vi "LC_Relay_main_WVM.vi"() -> ()   [LabVIEW 2016]
doc: "Reads relay data from FPGA layer. \nControls and coordinates all relays and relay functions. \nUses waveform data for measurements."
uses:
  <vilib>/Platform/TimedLoop/XDataNode/timing_clust.ctl
  <vilib>/Platform/TimedLoop/XDataNode/nitl_modes.ctl
  <vilib>/Platform/TimedLoop/XDataNode/wakeup.ctl
  <vilib>/FPGAPlugInAG/cRIO-9039 (Sync)/niLvFpga_Open_cRIO-9039 (Sync).vi
  <vilib>/rvi/interface/common/dynamic/niFpgaDynamicAddResources.vi
  <vilib>/Utility/error.llb/Error Cluster From Error Code.vi
  <vilib>/rvi/errors/niLvFpgaAdjustHostInterfaceError.vi
  <vilib>/FPGAPlugInAG/Dynamic/niLvFpga_Close_Dynamic.vi
  <vilib>/rvi/interface/nirviOpenFPGA/nirviOpenFPGA.xnode
  FPGA Bitfiles/IntelliRupter_calibrated.lvbitx
  <vilib>/rvi/interface/nirviReadWriteControl/nirviReadWriteControl.xnode
  <vilib>/Platform/TimedLoop/XDataNode/XDataNode.xnode
  <vilib>/rvi/interface/nirviCloseFPGA/nirviCloseFPGA.xnode
  <vilib>/rvi/interface/Simulation/niFpgaSimulationCallBeginRW.vi
  NiFpgaLv.dll
  <vilib>/Platform/TimedLoop/XDataNode/XDNodeRunTimeDep.lvlib
panel:
  in  "y 2":sgl=0.185
  out "basic calc interval":u16=2131
  out "half cycle (samples)":i32=96
  out "Waveform Chart 2":dbl(graph)=1.0951570390584209
  in  "I offset R2":dbl=-0.01
  in  "I offset R7":dbl
  in  "I offset R3":dbl=-0.12
  out "R8 Transfer":bool
  out "R7 Transfer":bool
  out "R5 Transfer":bool
  out "R4 Transfer":bool
  out "R2 Transfer":bool
  in  "I offset R8":dbl=0.09
  in  "I offset R4":dbl=0.02
  in  "I offset R6":dbl=0.09
  in  "I offset R5":dbl=0.03
  in  "I offset R1":dbl=-0.11
  in  "R8 Blocking in":bool
  in  "R7 Blocking in":bool
  in  "R6 Blocking in":bool
  in  "R5 Blocking in":bool
  in  "R4 Blocking in":bool
  in  "R3 Blocking in":bool
  in  "R2 Blocking in":bool
  in  "R1 Blocking in":bool
  out "R1 Blocking out":bool[](array[boolean])
  out "R2 Blocking out":bool[](array[boolean])
  out "R3 Blocking out":bool[](array[boolean])
  out "R4 Blocking out":bool[](array[boolean])
  out "R5 Blocking out":bool[](array[boolean])
  out "R6 Blocking out":bool[](array[boolean])
  out "R8 Blocking out":bool[](array[boolean])
  out "R7 Blocking out":bool[](array[boolean])
  out "Relay7 Reclose":bool=TRUE
  out "Relay7 Trip":bool
  out "Relay8 Reclose":bool=TRUE
  out "Relay8 Trip":bool
  out "Relay6 Reclose":bool=TRUE
  out "Relay6 Trip":bool
  out "Relay5 Reclose":bool=TRUE
  out "Relay5 Trip":bool
  out "Relay4 Reclose":bool=TRUE
  out "Relay4 Trip":bool
  out "Relay3 Reclose":bool=TRUE
  out "Relay3 Trip":bool
  out "Relay2 Reclose":bool=TRUE
  out "Relay2 Trip":bool
  out "Relay1 Reclose":bool=TRUE
  out "Relay1 Trip":bool
  in  "Manual Relay Control":bool
  out "Loop time":u32=60
  in  "Recloser Settings":T1={"Magnitude Minimum"=0.1, "Magnitude difference level"=0.05, "Frequency difference level"=0.02, "Phase difference level"=5.0}
  out "MGCC_to_relay":bool[](array[boolean])=[TRUE, TRUE, FALSE, FALSE, TRUE, TRUE, TRUE, TRUE]
  in  "Count(ticks)":u32=10000
  in  "RMS minimum\nvalues":cluster{"VRMS values":dbl, "IRMS values":dbl}={"VRMS values"=0.1, "IRMS values"=0.1}
  out "error out":errorcluster
  out "Relay_toMGCC":bool[](array[boolean])=[TRUE, TRUE, FALSE, FALSE, TRUE, TRUE, TRUE, TRUE]
  in  "Reclose Relay8?":bool=TRUE
  out "R8 Data for\ncommunication":dbl[](array[numeric])=[1.0, 0.9909150153075655, 0.9896188769976684, 63.47129196024821, 63.46582681259073, -0.5764253577681681, 0.09837072342634201, -0.0020060823298990726, 0.0, 0.0]
  in  "Reclose Relay7?":bool=TRUE
  out "R7 Data for\ncommunication":dbl[](array[numeric])=[1.0, 0.9922460509469712, 0.9943028155085312, 63.467411089646376, 63.478152065187864, -0.9460193616761975, -0.2064996361732483, -0.004409481305629015, 0.0, 0.0]
  in  "Reclose Relay6?":bool=TRUE
  out "R6 Data for\ncommunication":dbl[](array[numeric])=[1.0, 0.9915330670074546, 0.9917837391358869, 63.46965540740244, 63.478307865717966, -1.712720964622984, 0.09586220979690552, -0.0029444273095577955, 0.0, 0.0]
  in  "Reclose Relay5?":bool=TRUE
  out "R5 Data for\ncommunication":dbl[](array[numeric])=[1.0, 0.9909484160806271, 0.991066273342716, 63.47073917874258, 63.46653413553481, -1.6509056131861446, -0.0007275078096427023, -0.001496070297434926, 0.0, 0.0]
  in  "Reclose Relay4?":bool
  out "R4 Data for\ncommunication":dbl[](array[numeric])=[0.0, 0.9981886417791191, 0.9892796089659758, 61.74314245608404, 63.467147931305185, -104.14330841710972, 0.002056945115327835, 0.0013565359404310584, 0.0, 0.0]
  in  "Reclose Relay3?":bool
  out "R3 Data for\ncommunication":dbl[](array[numeric])=[0.0, 0.999365103685235, 1.047730543459152, 61.748556508686754, 61.74017682398038, 147.0934201296015, 0.0002776427718345076, -0.00020188414782751352, 0.0, 0.0]
  in  "Reclose Relay2?":bool=TRUE
  out "R2 Data for\ncommunication":dbl[](array[numeric])=[1.0, 0.9959757563522635, 0.9976363309245574, 61.748038041733366, 61.74666804059112, 1.0951570390584209, 0.08623241633176804, 0.03451136499643326, 0.0, -0.0013700011422486114]
  out "R1 Data for\ncommunication":dbl[](array[numeric])=[1.0, 0.9976265709226886, 0.9964869644913441, 61.738825153713954, 61.7422198127711, -0.049738413299934336, 0.18149961531162262, 0.06204972043633461, 0.0, 0.003394659057143201]
  in  "Relay8":bool=TRUE
  in  "Relay7":bool=TRUE
  in  "Relay6":bool=TRUE
  in  "Relay5":bool=TRUE
  in  "Relay4":bool
  in  "Relay3":bool
  in  "Relay2":bool=TRUE
  in  "Reclose Relay1?":bool=TRUE
  in  "stop":bool
  in  "Relay1":bool=TRUE
  # "status\nmag_left\nmag_right\nfreq_left\nfreq_right\nang_diff\nact_power\nrea_power\n0\n0"
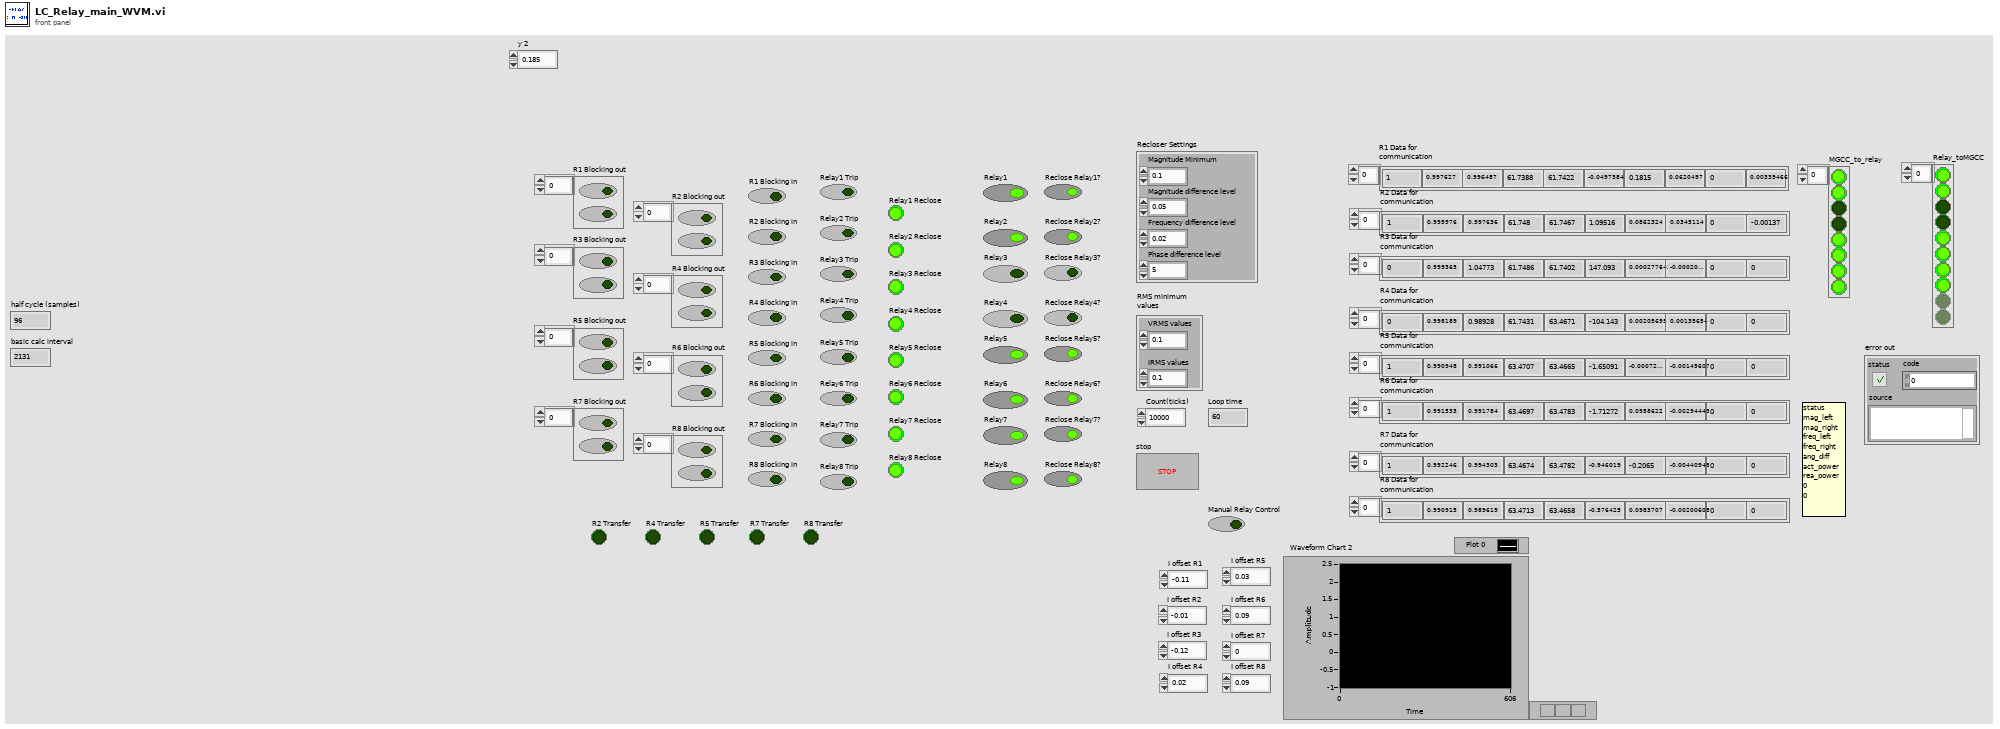
[diagram p1: front panel]
types:
  T1 = cluster{"Magnitude Minimum":dbl, "Magnitude difference level":dbl, "Frequency difference level":dbl, "Phase difference level":dbl}
  T2 = typedef "XDNodeRunTimeDep.lvlib/timing_clust.ctl" = cluster{"Expected End [f-1]":u64, "Actual End [f-1]":u64, "Finished Late? [f-1]":bool, "Expected End [i-1]":u64, "Actual End [i-1]":u64, "Finished Late? [i-1]":bool, "Expected Start [i]":u64, "Actual Start [i]":u64, "Expected Start [f]":u64, "Actual Start [f]":u64, "Source Name":string, "Structure Name":string, "Period":i64, "Deadline":i64, "Offset":i64, "Start":i64, "Priority":i32, "Timeout":i32, "Mode":T3, "Wakeup Reason":T4, "Error":errorcluster, "Source Type":string, "Secondary Source Type":string, "Global End Time":u64, "Global Start Time":u64, "Frame Duration":u64, "Iteration Duration":u64, "Assigned CPU":i32, "I/O Scan Engine Mode":u32}
  T3 = typedef "XDNodeRunTimeDep.lvlib/nitl_modes.ctl" = enum32{"No Change", "Process missed periods, maintain original phase", "Discard missed periods, maintain original phase", "Process missed periods, ignore original phase", "Discard missed periods, ignore original phase"}
  T4 = typedef "XDNodeRunTimeDep.lvlib/wakeup.ctl" = enum32{"Normal", "Aborted", "Asynchronous wakeup", "Timing source error", "Timed loop error", "Timeout"}
  T5 = enum16{"Grid-connected", "BESS only", "PV + BESS"}
  T6 = cluster{"UV Reset level":dbl, "Undervoltage \npick-up level":dbl, "OC Reset level":dbl, "Overcurrent\npick-up level":dbl, "time delay settings":cluster{"Definite operate time [ms]":u32, "Inverse Operating Time [ms]":u32, "reset time [ms]":u32, "operate time compensation [ms]":u32}}
  T7 = cluster{fxp<+/-,53,11>[], fxp<+/-,53,11>[], fxp<+/-,53,11>[], fxp<+/-,53,11>[], fxp<+/-,53,11>[], fxp<+/-,53,11>[], fxp<+/-,53,11>[], fxp<+/-,53,11>[], fxp<+/-,53,11>[]}
  T8 = typedef "NI_EP_Protection_FPGA.lvlib/fpga_Timer Feedback Var.ctl" = cluster{"time elapsed":u32, "start time of trip counting":u32, "start time of reseting":u32}
  T9 = typedef "NI_EP_Protection_FPGA.lvlib/fpga_State.ctl" = enum16{"Idle", "Trip Counting", "Tripped", "Reset Counting"}
  T10 = cluster{"Direction":enum16{"forward", "backward", "N/D"}, "Boolean":bool, "timing values out":T8, "status out":T9, "trip signal out":bool, "State Out":enum16{"Idle", "Wait for Trip", "PulseClosing", "Locked"}, "Pulse Index Out":i32, "start time of reseting":u32, bool}
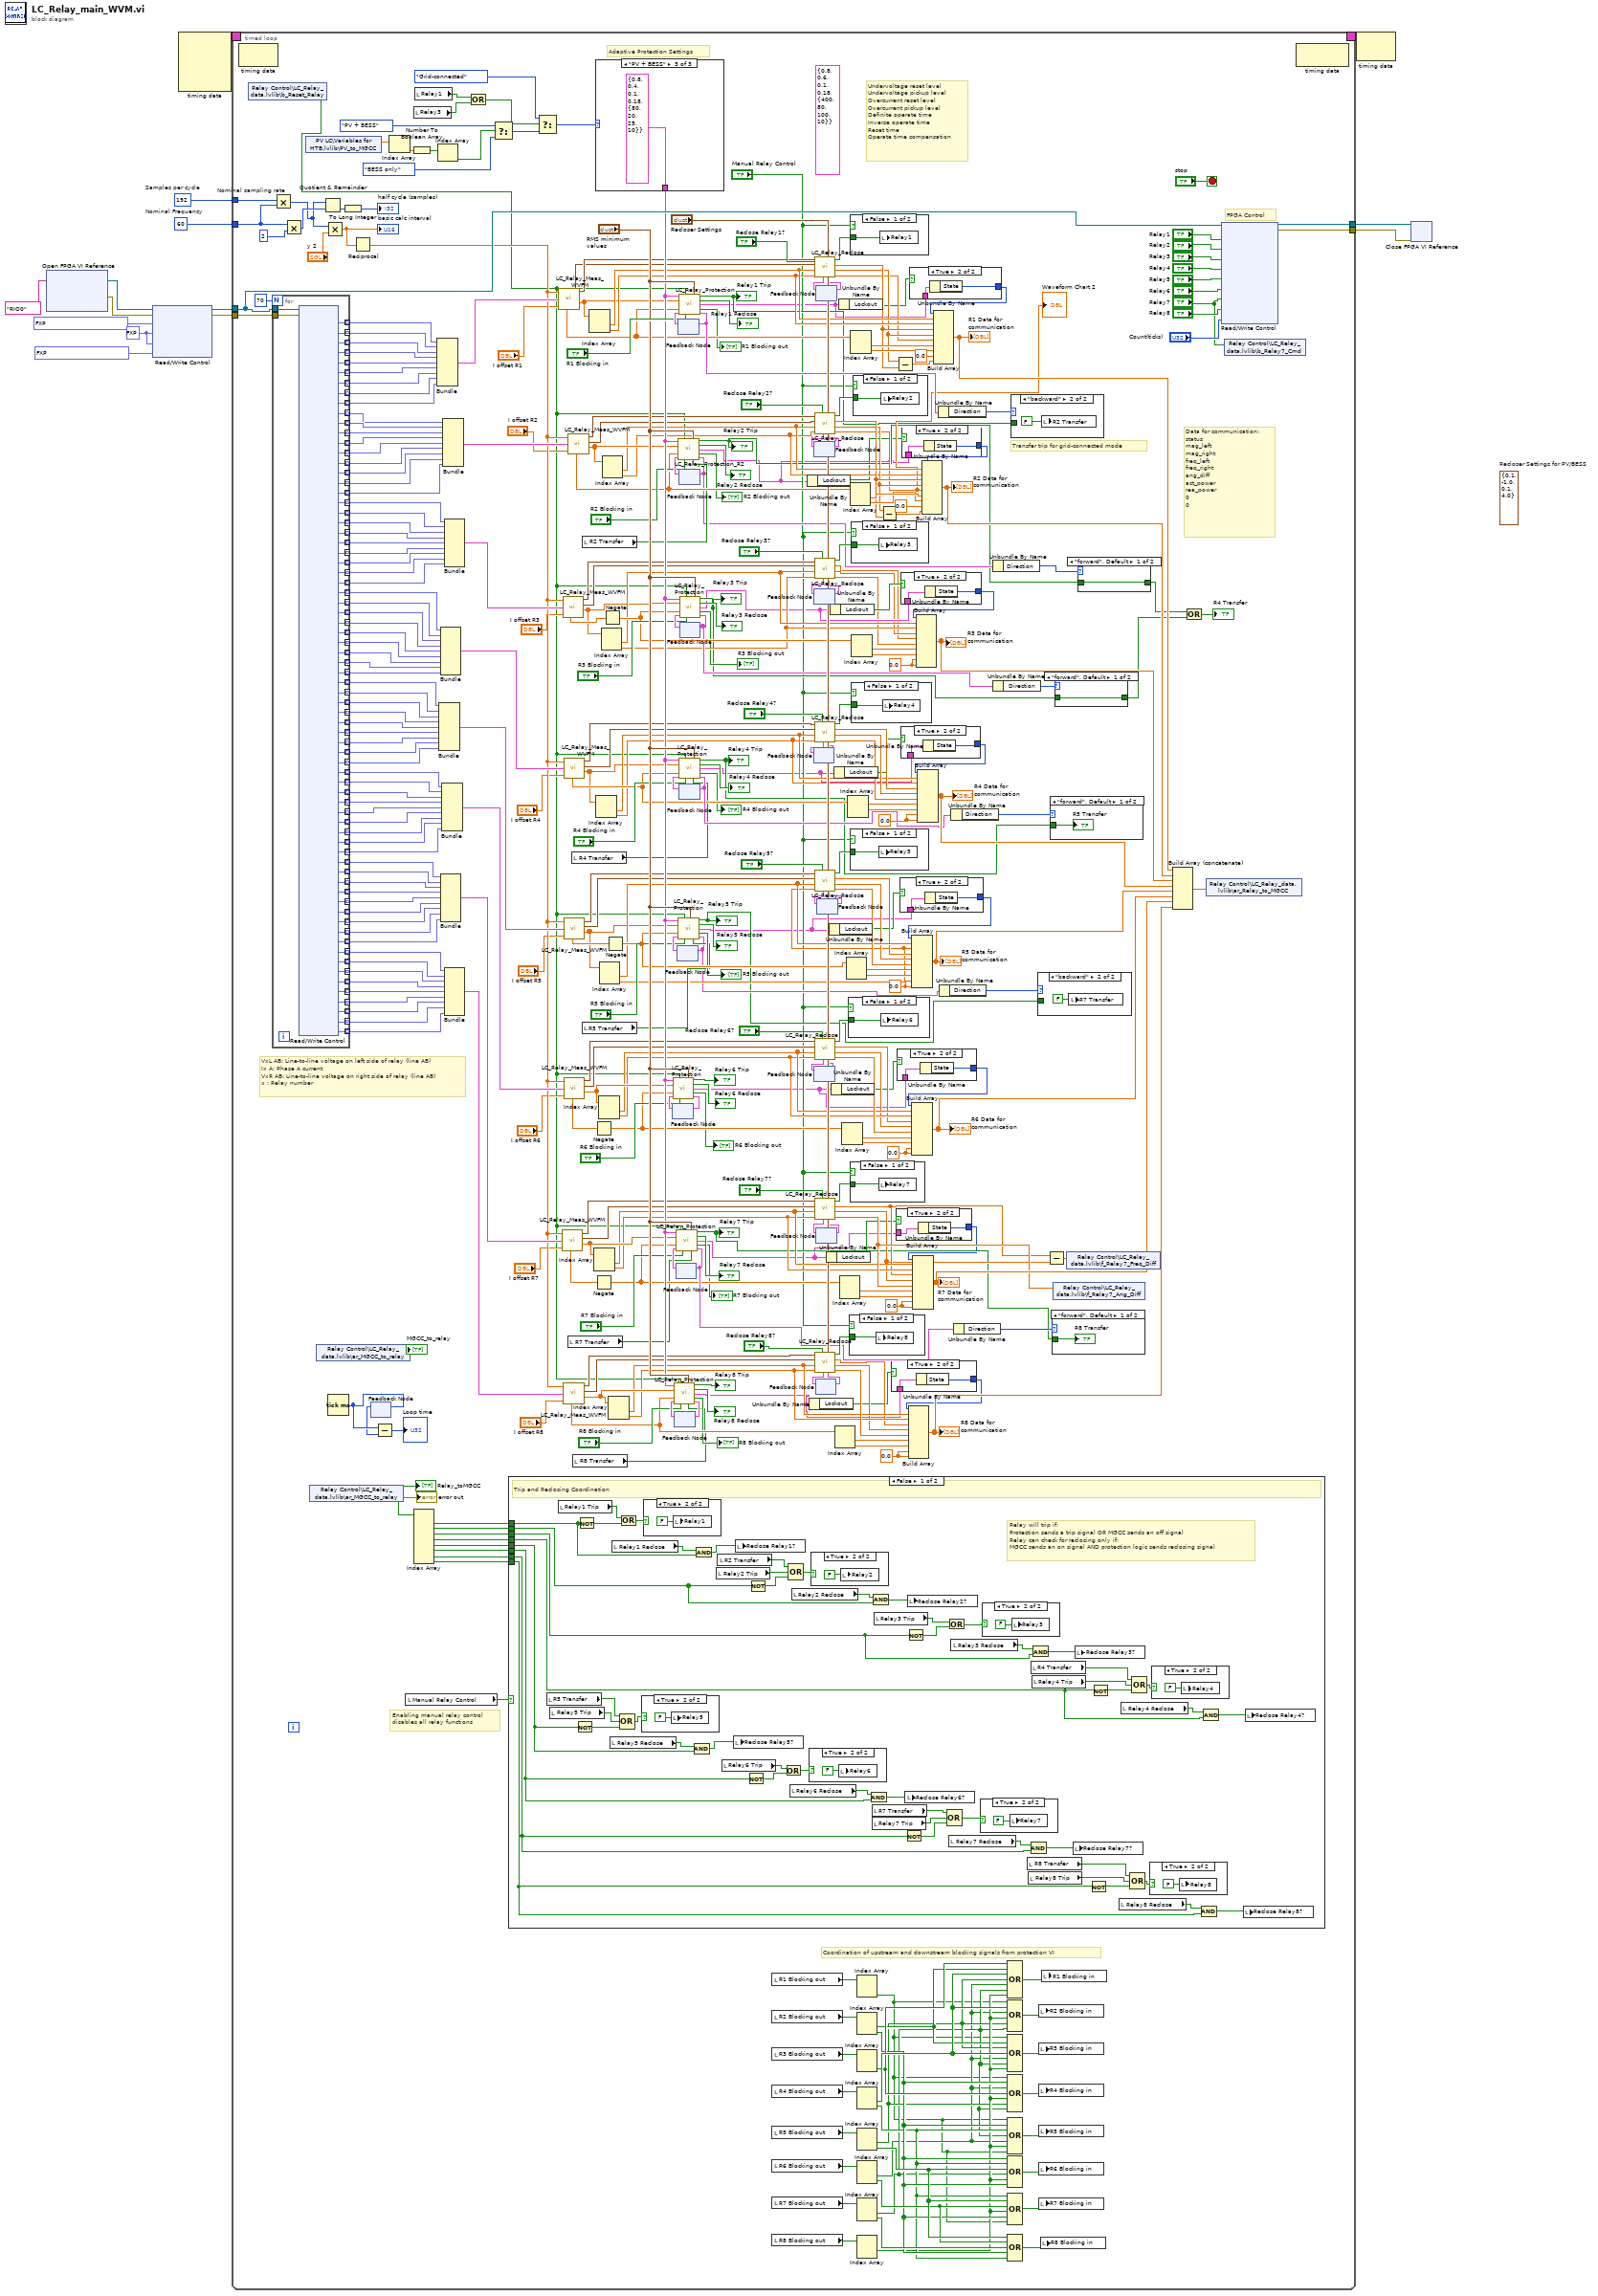
[diagram p0: block diagram]
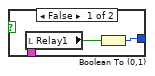
[diagram p2: hidden frame]
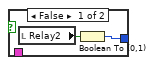
[diagram p3: hidden frame]
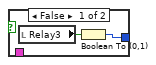
[diagram p4: hidden frame]
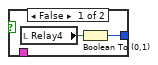
[diagram p5: hidden frame]
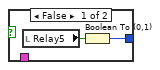
[diagram p6: hidden frame]
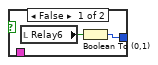
[diagram p7: hidden frame]
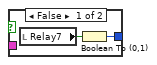
[diagram p8: hidden frame]
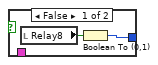
[diagram p9: hidden frame]
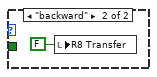
[diagram p10: hidden frame]
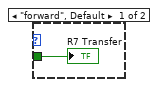
[diagram p11: hidden frame]
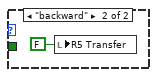
[diagram p12: hidden frame]
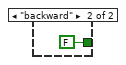
[diagram p13: hidden frame]
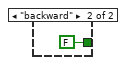
[diagram p14: hidden frame]
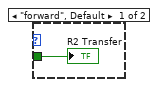
[diagram p15: hidden frame]
diagram:
  w2 = 192  # Samples per cycle
  w1 = 60  # Nominal Frequency
  (unwired) T1 {"Magnitude Minimum"=0.1, "Magnitude difference level"=-1.0, "Frequency difference level"=0.1, "Phase difference level"=4.0}  # Recloser Settings for PV/BESS
  w6 = fxp<+/-,52,10> 0.0 ("I offset")
  n1 = xnode "Open FPGA VI Reference"("resource name"=tag "RIO0") -> ("FPGA VI Reference Out"=w5:refnum<k20>, "error out"=w10:errorcluster)  [unwired: 1 in]
  n2 = xnode "Read/Write Control"("FPGA VI Reference In"=w5, "error in"=w10, "I scale factor"=fxp<+/-,26,5> 0.4850001335144043, "I offset"=w6, "V offset"=w6, "V scale factor"=fxp<+/-,26,5> 0.40000009536743164) -> ("FPGA VI Reference Out"=w11:refnum<k20>, "error out"=w9:errorcluster)
  n3 = node-c288() -> (w4:T2)  [unwired: 4 in]
  n4 = timed-loop {
    tunnel: w11 -> [w415]
    tunnel: [w417] -> w13
    tunnel: [w416] -> w12
    tunnel: w9 -> [w414]
    timing: w4 -> [_]
    timing-out: [_] -> w3
    tunnel: w2 -> [w121]
    tunnel: w1 -> [w120]
    stop <- "stop" stop-if-true
    (unwired) T6 {"UV Reset level"=0.8, "Undervoltage \npick-up level"=0.6, "OC Reset level"=0.1, "Overcurrent\npick-up level"=0.18, "time delay settings"={"Definite operate time [ms]"=400, "Inverse Operating Time [ms]"=80, "reset time [ms]"=100, "operate time compensation [ms]"=10}} ("Protection settings")
    w269 = 0.0 ("element")
    w270 = 0.0 ("element")
    w279 = 0.0 ("element")
    w162 = 0.0 ("element")
    w289 = 0.0 ("element")
    w290 = 0.0 ("element")
    # "Enabling manual relay control \ndisables all relay functions"
    # "Coordination of upstream and downstream blocking signals from protection VI"
    # "VxL AB: Line-to-line voltage on left side of relay (line AB)\nIx A: Phase A current\nVxR AB: Line-to-line voltage on right side of relay (line AB)\nx : Relay number"
    # "FPGA Control"
    # "Transfer trip for grid-connected mode"
    # "Undervoltage reset level\nUndervoltage pickup level\nOvercurrent reset level\nOvercurrent pickup level\nDefinite operate time\nInverse operate time\nReset time\nOperate time compensation"
    # "Adaptive Protection Settings"
    # "Data for communication:\nstatus\nmag_left\nmag_right\nfreq_left\nfreq_right\nang_diff\nact_power\nrea_power\n0\n0"
    n5 = node-c288() -> ()  [unwired: 1 in, 1 out]
    n6 = shared-variable "Relay Control\\LC_Relay_data.lvlib\\b_Reset_Relay"() -> (w25:bool)  [unwired: 1 in, 1 out]
    n7 = for {
      N: 70 -> [_]
      tunnel: w415 -> [w524]
      tunnel: w414 -> [w523]
      tunnel: [w522] -> w413 mode=indexing
      tunnel: [w521] -> w412 mode=indexing
      tunnel: [w520] -> w411 mode=indexing
      tunnel: [w519] -> w410 mode=indexing
      tunnel: [w518] -> w409 mode=indexing
      tunnel: [w517] -> w408 mode=indexing
      tunnel: [w516] -> w407 mode=indexing
      tunnel: [w515] -> w406 mode=indexing
      tunnel: [w514] -> w24 mode=indexing
      tunnel: [w513] -> w22 mode=indexing
      tunnel: [w512] -> w21 mode=indexing
      tunnel: [w511] -> w20 mode=indexing
      tunnel: [w510] -> w19 mode=indexing
      tunnel: [w509] -> w18 mode=indexing
      tunnel: [w508] -> w395 mode=indexing
      tunnel: [w507] -> w394 mode=indexing
      tunnel: [w506] -> w393 mode=indexing
      tunnel: [w505] -> w392 mode=indexing
      tunnel: [w504] -> w391 mode=indexing
      tunnel: [w503] -> w390 mode=indexing
      tunnel: [w502] -> w389 mode=indexing
      tunnel: [w501] -> w388 mode=indexing
      tunnel: [w500] -> w387 mode=indexing
      tunnel: [w499] -> w386 mode=indexing
      tunnel: [w498] -> w385 mode=indexing
      tunnel: [w497] -> w384 mode=indexing
      tunnel: [w496] -> w383 mode=indexing
      tunnel: [w495] -> w382 mode=indexing
      tunnel: [w494] -> w381 mode=indexing
      tunnel: [w493] -> w380 mode=indexing
      tunnel: [w492] -> w379 mode=indexing
      tunnel: [w491] -> w378 mode=indexing
      tunnel: [w490] -> w377 mode=indexing
      tunnel: [w489] -> w376 mode=indexing
      tunnel: [w488] -> w375 mode=indexing
      tunnel: [w487] -> w374 mode=indexing
      tunnel: [w486] -> w373 mode=indexing
      tunnel: [w485] -> w372 mode=indexing
      tunnel: [w484] -> w371 mode=indexing
      tunnel: [w483] -> w370 mode=indexing
      tunnel: [w482] -> w369 mode=indexing
      tunnel: [w481] -> w368 mode=indexing
      tunnel: [w480] -> w367 mode=indexing
      tunnel: [w479] -> w366 mode=indexing
      tunnel: [w478] -> w365 mode=indexing
      tunnel: [w477] -> w364 mode=indexing
      tunnel: [w476] -> w363 mode=indexing
      tunnel: [w475] -> w362 mode=indexing
      tunnel: [w474] -> w361 mode=indexing
      tunnel: [w473] -> w360 mode=indexing
      tunnel: [w472] -> w359 mode=indexing
      tunnel: [w471] -> w358 mode=indexing
      tunnel: [w470] -> w357 mode=indexing
      tunnel: [w469] -> w356 mode=indexing
      tunnel: [w468] -> w355 mode=indexing
      tunnel: [w467] -> w354 mode=indexing
      tunnel: [w466] -> w353 mode=indexing
      tunnel: [w465] -> w352 mode=indexing
      tunnel: [w464] -> w351 mode=indexing
      tunnel: [w463] -> w350 mode=indexing
      tunnel: [w462] -> w349 mode=indexing
      tunnel: [w461] -> w348 mode=indexing
      tunnel: [w460] -> w299 mode=indexing
      tunnel: [w459] -> w23 mode=indexing
      tunnel: [w458] -> w217 mode=indexing
      tunnel: [w457] -> w216 mode=indexing
      tunnel: [w456] -> w215 mode=indexing
      tunnel: [w455] -> w214 mode=indexing
      tunnel: [w454] -> w213 mode=indexing
      tunnel: [w453] -> w212 mode=indexing
      tunnel: [w452] -> w211 mode=indexing
      tunnel: [w451] -> w210 mode=indexing
      n8 = xnode "Read/Write Control"("FPGA VI Reference In"=w524, "error in"=w523) -> ("V1L AB"=w460:fxp<+/-,53,11>, "V1L BC"=w522:fxp<+/-,53,11>, "V1L CA"=w521:fxp<+/-,53,11>, "V1R AB"=w520:fxp<+/-,53,11>, "V1R BC"=w519:fxp<+/-,53,11>, "V1R CA"=w518:fxp<+/-,53,11>, "I1 A"=w517:fxp<+/-,53,11>, "I1 B"=w516:fxp<+/-,53,11>, "I1 C"=w515:fxp<+/-,53,11>, "V2L AB"=w459:fxp<+/-,53,11>, "V2L BC"=w458:fxp<+/-,53,11>, "V2L CA"=w457:fxp<+/-,53,11>, "V2R AB"=w456:fxp<+/-,53,11>, "V2R BC"=w455:fxp<+/-,53,11>, "V2R CA"=w454:fxp<+/-,53,11>, "I2 A"=w453:fxp<+/-,53,11>, "I2 B"=w452:fxp<+/-,53,11>, "I2 C"=w451:fxp<+/-,53,11>, "V3L AB"=w514:fxp<+/-,53,11>, "V3L BC"=w513:fxp<+/-,53,11>, "V3L CA"=w512:fxp<+/-,53,11>, "V3R AB"=w511:fxp<+/-,53,11>, "V3R BC"=w510:fxp<+/-,53,11>, "V3R CA"=w509:fxp<+/-,53,11>, "I3 A"=w508:fxp<+/-,53,11>, "I3 B"=w507:fxp<+/-,53,11>, "I3 C"=w506:fxp<+/-,53,11>, "V4L AB"=w505:fxp<+/-,53,11>, "V4L BC"=w504:fxp<+/-,53,11>, "V4L CA"=w503:fxp<+/-,53,11>, "V4R AB"=w502:fxp<+/-,53,11>, "V4R BC"=w501:fxp<+/-,53,11>, "V4R CA"=w500:fxp<+/-,53,11>, "I4 A"=w499:fxp<+/-,53,11>, "I4 B"=w498:fxp<+/-,53,11>, "I4 C"=w497:fxp<+/-,53,11>, "V5L AB"=w496:fxp<+/-,53,11>, "V5L BC"=w495:fxp<+/-,53,11>, "V5L CA"=w494:fxp<+/-,53,11>, "V5R AB"=w493:fxp<+/-,53,11>, "V5R BC"=w492:fxp<+/-,53,11>, "V5R CA"=w491:fxp<+/-,53,11>, "I5 A"=w490:fxp<+/-,53,11>, "I5 B"=w489:fxp<+/-,53,11>, "I5 C"=w488:fxp<+/-,53,11>, "V6L AB"=w487:fxp<+/-,53,11>, "V6L BC"=w486:fxp<+/-,53,11>, "V6L CA"=w485:fxp<+/-,53,11>, "V6R AB"=w484:fxp<+/-,53,11>, "V6R BC"=w483:fxp<+/-,53,11>, "V6R CA"=w482:fxp<+/-,53,11>, "I6 A"=w481:fxp<+/-,53,11>, "I6 B"=w480:fxp<+/-,53,11>, "I6 C"=w479:fxp<+/-,53,11>, "V7L AB"=w478:fxp<+/-,53,11>, "V7L BC"=w477:fxp<+/-,53,11>, "V7L CA"=w476:fxp<+/-,53,11>, "V7R AB"=w475:fxp<+/-,53,11>, "V7R BC"=w474:fxp<+/-,53,11>, "V7R CA"=w473:fxp<+/-,53,11>, "I7 A"=w472:fxp<+/-,53,11>, "I7 B"=w471:fxp<+/-,53,11>, "I7 C"=w470:fxp<+/-,53,11>, "V8L AB"=w469:fxp<+/-,53,11>, "V8L BC"=w468:fxp<+/-,53,11>, "V8L CA"=w467:fxp<+/-,53,11>, "V8R AB"=w466:fxp<+/-,53,11>, "V8R BC"=w465:fxp<+/-,53,11>, "V8R CA"=w464:fxp<+/-,53,11>, "I8 A"=w463:fxp<+/-,53,11>, "I8 B"=w462:fxp<+/-,53,11>, "I8 C"=w461:fxp<+/-,53,11>)  [unwired: 2 out]
    }
    n9 = Multiply "Nominal sampling rate"(x=w121, y=w120) -> (x*y=w123:i32)
    n10 = Multiply(x=w120, y=2) -> (x*y=w127:i32)
    n11 = shared-variable "PV LC\\Variables for HTB.lvlib\\PV_to_MGCC"() -> (w109:dbl[])  [unwired: 1 in, 1 out]
    n12 = shared-variable "Relay Control\\LC_Relay_data.lvlib\\ar_MGCC_to_relay"() -> (w335:bool[], error out=→"error out":errorcluster)  [unwired: 1 in]
    "Relay_toMGCC" <- w335
    n13 = shared-variable "Relay Control\\LC_Relay_data.lvlib\\ar_MGCC_to_relay"() -> (→"MGCC_to_relay":bool[])  [unwired: 1 in, 1 out]
    n14 = Quotient & Remainder(x=w123, y=w127) -> (floor(x/y)=w125:i32)  [unwired: 1 out]
    n15 = Multiply(x=w123, y="y 2") -> (x*y=w122:sgl)
    "basic calc interval" <- w122
    n16 = Tick Count (ms)() -> (millisecond timer value=w327:u32)
    n17 = To Long Integer(number=w125) -> (32bit integer=→"half cycle (samples)":i32)
    n18 = Reciprocal(x=w122) -> (1/x=w119:sgl)
    n19 = feedback #1() -> (w326:u32)  [unwired: 1 in]
    n20 = feedback-in #1(w327) -> ()
    n21 = Subtract(x=w327, y=w326) -> (x-y=→"Loop time":u32)
    n22 = Index Array(array=w109) -> (element=w332:dbl)  [unwired: 1 in]
    n23 = local read "Manual Relay Control"() -> (w307:bool)
    n24 = Number To Boolean Array(number=w332) -> (Boolean array=w331:bool[])
    n25 = local read "Relay3"() -> (w58:bool)
    n26 = Index Array(array=w335) -> (element #1=w315:bool, element #2=w314:bool, element #3=w313:bool, element #4=w312:bool, element #5=w311:bool, element #6=w310:bool, element #7=w309:bool, element #8=w308:bool)  [unwired: 8 in]
    n27 = local read "Relay1"() -> (w59:bool)
    n28 = Bundle(w299, w413, w412, w411, w410, w409, w408, w407, w406) -> (w205:T7)  [unwired: 1 in]
    n29 = Index Array(array=w331) -> (element=w330:bool)  [unwired: 1 in]
    n30 = Bundle(w383, w382, w381, w380, w379, w378, w377, w376, w375) -> (w322:T7)  [unwired: 1 in]
    n31 = Bundle(w392, w391, w390, w389, w388, w387, w386, w385, w384) -> (w323:T7)  [unwired: 1 in]
    n32 = Bundle(w365, w364, w363, w362, w361, w360, w359, w358, w357) -> (w320:T7)  [unwired: 1 in]
    n33 = Bundle(w374, w373, w372, w371, w370, w369, w368, w367, w366) -> (w321:T7)  [unwired: 1 in]
    n34 = Bundle(w23, w217, w216, w215, w214, w213, w212, w211, w210) -> (w209:T7)  [unwired: 1 in]
    n35 = Bundle(w24, w22, w21, w20, w19, w18, w395, w394, w393) -> (w324:T7)  [unwired: 1 in]
    n36 = Bundle(w356, w355, w354, w353, w352, w351, w350, w349, w348) -> (w319:T7)  [unwired: 1 in]
    n37 = Or(x=w59, y=w58) -> (x .or. y?=w57:bool)
    n38 = Select(t=T5."PV + BESS", s=w330, f=T5."BESS only") -> (s? t:f=w60:T5)
    n39 = case shown="False" w307 {
      tunnel: w315 -> [w584 _]
      tunnel: w314 -> [w582 _]
      tunnel: w313 -> [w578 _]
      tunnel: w312 -> [w575 _]
      tunnel: w311 -> [w554 _]
      tunnel: w310 -> [w553 _]
      tunnel: w309 -> [w552 _]
      tunnel: w308 -> [w551 _]
      frame False {
        # "Relay will trip if:\nProtection sends a trip signal OR MGCC sends an off signal\nRelay can check for reclosing only if:\nMGCC sends an on signal AND protection logic sends reclosing signal"
        # "Trip and Reclosing Coordination"
        n40 = local read "R5 Transfer"() -> (w548:bool)
        n41 = local read "Relay5 Trip"() -> (w555:bool)
        n42 = local read "Relay1 Trip"() -> (w598:bool)
        n43 = Not(x=w554) -> (.not. x?=w557:bool)
        n44 = Not(x=w584) -> (.not. x?=w596:bool)
        n45 = local read "Relay5 Reclose"() -> (w568:bool)
        n46 = local read "Relay1 Reclose"() -> (w585:bool)
        n47 = Or(x=w598, y=w596) -> (x .or. y?=w597:bool)
        n48 = Compound Arithmetic op=OR(w548, w555, w557) -> (w556:bool)
        n49 = case shown="True" w556 {
          frame False {
          }
          frame True {
            n50 = local write "Relay5"(FALSE ("Relay8")) -> ()
          }
        }
        n51 = case shown="True" w597 {
          frame False {
          }
          frame True {
            n52 = local write "Relay1"(FALSE ("Relay8")) -> ()
          }
        }
        n53 = And(x=w585, y=w584) -> (x .and. y?=w586:bool)
        n54 = Compound Arithmetic op=AND(w568, w554) -> (w567:bool)
        n55 = local read "Relay2 Trip"() -> (w589:bool)
        n56 = local read "R2 Transfer"() -> (w550:bool)
        n57 = local read "Relay6 Trip"() -> (w564:bool)
        n58 = local write "Reclose Relay5?"(w567) -> ()
        n59 = local write "Reclose Relay1?"(w586) -> ()
        n60 = Not(x=w553) -> (.not. x?=w558:bool)
        n61 = Not(x=w582) -> (.not. x?=w595:bool)
        n62 = Or(x=w564, y=w558) -> (x .or. y?=w559:bool)
        n63 = Compound Arithmetic op=OR(w550, w589, w595) -> (w594:bool)
        n64 = local read "Relay6 Reclose"() -> (w570:bool)
        n65 = local read "Relay2 Reclose"() -> (w581:bool)
        n66 = case shown="True" w559 {
          frame False {
          }
          frame True {
            n67 = local write "Relay6"(FALSE ("Relay8")) -> ()
          }
        }
        n68 = case shown="True" w594 {
          frame False {
          }
          frame True {
            n69 = local write "Relay2"(FALSE ("Relay8")) -> ()
          }
        }
        n70 = And(x=w570, y=w553) -> (x .and. y?=w569:bool)
        n71 = local read "R7 Transfer"() -> (w547:bool)
        n72 = local read "Relay7 Trip"() -> (w565:bool)
        n73 = Compound Arithmetic op=AND(w581, w582) -> (w583:bool)
        n74 = local read "Relay3 Trip"() -> (w588:bool)
        n75 = Not(x=w552) -> (.not. x?=w561:bool)
        n76 = local write "Reclose Relay6?"(w569) -> ()
        n77 = Not(x=w578) -> (.not. x?=w592:bool)
        n78 = local write "Reclose Relay2?"(w583) -> ()
        n79 = Or(x=w588, y=w592) -> (x .or. y?=w593:bool)
        n80 = Compound Arithmetic op=OR(w547, w565, w561) -> (w560:bool)
        n81 = local read "Relay7 Reclose"() -> (w572:bool)
        n82 = local read "Relay3 Reclose"() -> (w579:bool)
        n83 = case shown="True" w560 {
          frame False {
          }
          frame True {
            n84 = local write "Relay7"(FALSE ("Relay8")) -> ()
          }
        }
        n85 = case shown="True" w593 {
          frame False {
          }
          frame True {
            n86 = local write "Relay3"(FALSE ("Relay8")) -> ()
          }
        }
        n87 = local read "R8 Transfer"() -> (w546:bool)
        n88 = local read "Relay8 Trip"() -> (w566:bool)
        n89 = And(x=w579, y=w578) -> (x .and. y?=w580:bool)
        n90 = local read "R4 Transfer"() -> (w549:bool)
        n91 = Compound Arithmetic op=AND(w572, w552) -> (w571:bool)
        n92 = local read "Relay4 Trip"() -> (w587:bool)
        n93 = local write "Reclose Relay7?"(w571) -> ()
        n94 = local write "Reclose Relay3?"(w580) -> ()
        n95 = Not(x=w551) -> (.not. x?=w562:bool)
        n96 = Not(x=w575) -> (.not. x?=w591:bool)
        n97 = local read "Relay8 Reclose"() -> (w573:bool)
        n98 = local read "Relay4 Reclose"() -> (w577:bool)
        n99 = Compound Arithmetic op=OR(w546, w566, w562) -> (w563:bool)
        n100 = Compound Arithmetic op=OR(w549, w587, w591) -> (w590:bool)
        n101 = case shown="True" w563 {
          frame False {
          }
          frame True {
            n102 = local write "Relay8"(FALSE ("Relay8")) -> ()
          }
        }
        n103 = case shown="True" w590 {
          frame False {
          }
          frame True {
            n104 = local write "Relay4"(FALSE ("Relay8")) -> ()
          }
        }
        n105 = Compound Arithmetic op=AND(w573, w551) -> (w574:bool)
        n106 = Compound Arithmetic op=AND(w577, w575) -> (w576:bool)
        n107 = local write "Reclose Relay8?"(w574) -> ()
        n108 = local write "Reclose Relay4?"(w576) -> ()
      }
      frame True {
      }
    }
    n109 = Select(t=T5."Grid-connected", s=w57, f=w60) -> (s? t:f=w61:T5)
    n110 = call "LC_Relay_Meas_WVFM.vi"("dt"=w119, "Input cluster"=w205, "Ioffset"="I offset R1") -> ("Total power values"=w191:dbl[], "VL array"=w201:waveform(sgl)[], "VR array"=w200:waveform(sgl)[], "RMS values"=w195:dbl[])  [unwired: 1 in, 1 out]
    n111 = call "LC_Relay_Meas_WVFM.vi"("dt"=w119, "Input cluster"=w320, "Ioffset"="I offset R7") -> ("Total power values"=w146:dbl[], "VL array"=w145:waveform(sgl)[], "VR array"=w144:waveform(sgl)[], "RMS values"=w143:dbl[])  [unwired: 1 in, 1 out]
    n112 = call "LC_Relay_Meas_WVFM.vi"("dt"=w119, "Input cluster"=w324, "Ioffset"="I offset R3") -> ("Total power values"=w179:dbl[], "VL array"=w181:waveform(sgl)[], "VR array"=w180:waveform(sgl)[], "RMS values"=w157:dbl[])  [unwired: 1 in, 1 out]
    n113 = call "LC_Relay_Meas_WVFM.vi"("dt"=w119, "Input cluster"=w319, "Ioffset"="I offset R8") -> ("Total power values"=w138:dbl[], "VL array"=w137:waveform(sgl)[], "VR array"=w136:waveform(sgl)[], "RMS values"=w135:dbl[])  [unwired: 1 in, 1 out]
    n114 = call "LC_Relay_Meas_WVFM.vi"("dt"=w119, "Input cluster"=w323, "Ioffset"="I offset R4") -> ("Total power values"=w175:dbl[], "VL array"=w171:waveform(sgl)[], "VR array"=w172:waveform(sgl)[], "RMS values"=w158:dbl[])  [unwired: 1 in, 1 out]
    n115 = call "LC_Relay_Meas_WVFM.vi"("dt"=w119, "Input cluster"=w322, "Ioffset"="I offset R5") -> ("Total power values"=w164:dbl[], "VL array"=w166:waveform(sgl)[], "VR array"=w165:waveform(sgl)[], "RMS values"=w159:dbl[])  [unwired: 1 in, 1 out]
    n116 = call "LC_Relay_Meas_WVFM.vi"("dt"=w119, "Input cluster"=w321, "Ioffset"="I offset R6") -> ("Total power values"=w156:dbl[], "VL array"=w154:waveform(sgl)[], "VR array"=w153:waveform(sgl)[], "RMS values"=w155:dbl[])  [unwired: 1 in, 1 out]
    n117 = call "LC_Relay_Meas_WVFM.vi"("dt"=w119, "Input cluster"=w209, "Ioffset"="I offset R2") -> ("Total power values"=w190:dbl[], "VL array"=w193:waveform(sgl)[], "VR array"=w192:waveform(sgl)[], "RMS values"=w189:dbl[])  [unwired: 1 in, 1 out]
    n118 = local read "R7 Transfer"() -> (w99:bool)
    n119 = local read "R4 Transfer"() -> (w97:bool)
    n120 = local read "R8 Transfer"() -> (w100:bool)
    n121 = local read "R5 Transfer"() -> (w98:bool)
    n122 = local read "R2 Transfer"() -> (w96:bool)
    n123 = Index Array(array=w195) -> (element #1=w199:dbl, element #2=w198:dbl)  [unwired: 2 in]
    n124 = Negate(x=w156) -> (-x=w219:dbl[])
    n125 = Index Array(array=w143) -> (element #1=w142:dbl, element #2=w141:dbl)  [unwired: 2 in]
    n126 = Negate(x=w146) -> (-x=w218:dbl[])
    n127 = case shown="\"PV + BESS\"" w61 {
      tunnel: [T6 {"UV Reset level"=0.9, "Undervoltage \npick-up level"=0.8, "OC Reset level"=0.1, "Overcurrent\npick-up level"=0.5, "time delay settings"={"Definite operate time [ms]"=400, "Inverse Operating Time [ms]"=100, "reset time [ms]"=100, "operate time compensation [ms]"=10}} ("Protection settings") T6 {"UV Reset level"=0.7, "Undervoltage \npick-up level"=0.5, "OC Reset level"=0.1, "Overcurrent\npick-up level"=0.17, "time delay settings"={"Definite operate time [ms]"=200, "Inverse Operating Time [ms]"=45, "reset time [ms]"=100, "operate time compensation [ms]"=10}} ("Protection settings") T6 {"UV Reset level"=0.8, "Undervoltage \npick-up level"=0.4, "OC Reset level"=0.1, "Overcurrent\npick-up level"=0.18, "time delay settings"={"Definite operate time [ms]"=80, "Inverse Operating Time [ms]"=20, "reset time [ms]"=25, "operate time compensation [ms]"=10}} ("Protection settings")] -> w303
      frame "Grid-connected", Default {
      }
      frame "BESS only" {
      }
      frame "PV + BESS" {
      }
    }
    n128 = Index Array(array=w158) -> (element #1=w170:dbl, element #2=w169:dbl)  [unwired: 2 in]
    n129 = Index Array(array=w155) -> (element #1=w150:dbl, element #2=w149:dbl)  [unwired: 2 in]
    n130 = Index Array(array=w159) -> (element #1=w163:dbl, element #2=w93:dbl)  [unwired: 2 in]
    n131 = Index Array(array=w157) -> (element #1=w183:dbl, element #2=w182:dbl)  [unwired: 2 in]
    n132 = Index Array(array=w189) -> (element #1=w188:dbl, element #2=w94:dbl)  [unwired: 2 in]
    n133 = Negate(x=w179) -> (-x=w228:dbl[])
    n134 = Negate(x=w164) -> (-x=w230:dbl[])
    n135 = Index Array(array=w135) -> (element #1=w132:dbl, element #2=w131:dbl)  [unwired: 2 in]
    n136 = feedback #2() -> (w256:T10)  [unwired: 1 in]
    n137 = call "LC_Relay_Protection.vi"("Protection settings"=w303, "Reset Relay"=w25, "RMS minimum\nvalues"="RMS minimum\nvalues", "RMS values"=w155, "Total power values"=w219, "input cluster"=w256, "Blocking in"="R6 Blocking in") -> ("trip signal"=→"Relay6 Trip":bool, "Reclose"=→"Relay6 Reclose":bool, "Relay State"=w30:cluster{"Lockout":bool, "State":i16}, "Blocking out"=→"R6 Blocking out":bool[], "output cluster"=w257:T10)  [unwired: 3 in, 1 out]
    n138 = feedback-in #2(w257) -> ()
    n139 = feedback #3() -> (w253:T10)  [unwired: 1 in]
    n140 = call "LC_Relay_Protection.vi"("Protection settings"=w303, "Reset Relay"=w25, "RMS minimum\nvalues"="RMS minimum\nvalues", "RMS values"=w135, "Total power values"=w138, "input cluster"=w253, "Blocking in"="R8 Blocking in", "Transfer Trip"=w100) -> ("trip signal"=→"Relay8 Trip":bool, "Reclose"=→"Relay8 Reclose":bool, "Relay State"=w28:cluster{"Lockout":bool, "State":i16}, "Blocking out"=→"R8 Blocking out":bool[], "output cluster"=w254:T10)  [unwired: 2 in, 1 out]
    n141 = feedback-in #3(w254) -> ()
    n142 = feedback #4() -> (w255:T10)  [unwired: 1 in]
    n143 = call "LC_Relay_Protection.vi"("Protection settings"=w303, "Reset Relay"=w25, "RMS minimum\nvalues"="RMS minimum\nvalues", "RMS values"=w143, "Total power values"=w218, "input cluster"=w255, "Blocking in"="R7 Blocking in", "Transfer Trip"=w99) -> ("trip signal"=w50:bool, "Reclose"=→"Relay7 Reclose":bool, "Relay State"=w29:cluster{"Lockout":bool, "State":i16}, "Blocking out"=→"R7 Blocking out":bool[], "output cluster"=w221:T10)  [unwired: 2 in, 1 out]
    "Relay7 Trip" <- w50
    n144 = feedback-in #4(w221) -> ()
    n145 = feedback #5() -> (w233:T10)  [unwired: 1 in]
    n146 = feedback #6() -> (w317:T10)  [unwired: 1 in]
    n147 = call "LC_Relay_Protection.vi"("Protection settings"=w303, "Reset Relay"=w25, "RMS minimum\nvalues"="RMS minimum\nvalues", "RMS values"=w159, "Total power values"=w230, "input cluster"=w233, "Blocking in"="R5 Blocking in", "Transfer Trip"=w98) -> ("trip signal"=w48:bool, "Reclose"=→"Relay5 Reclose":bool, "Relay State"=w31:cluster{"Lockout":bool, "State":i16}, "Blocking out"=→"R5 Blocking out":bool[], "output cluster"=w91:T10)  [unwired: 2 in, 1 out]
    "Relay5 Trip" <- w48
    n148 = feedback-in #5(w91) -> ()
    n149 = call "LC_Relay_Protection.vi"("Protection settings"=w303, "Reset Relay"=w25, "RMS minimum\nvalues"="RMS minimum\nvalues", "RMS values"=w195, "Total power values"=w191, "input cluster"=w317, "Blocking in"="R1 Blocking in") -> ("trip signal"=w44:bool, "Reclose"=→"Relay1 Reclose":bool, "Relay State"=w40:cluster{"Lockout":bool, "State":i16}, "Blocking out"=→"R1 Blocking out":bool[], "output cluster"=w302:T10)  [unwired: 3 in, 1 out]
    "Relay1 Trip" <- w44
    n150 = feedback-in #6(w302) -> ()
    n151 = feedback #7() -> (w259:T10)  [unwired: 1 in]
    n152 = call "LC_Relay_Protection_R2.vi"("Protection settings"=w303, "Reset Relay"=w25, "RMS minimum\nvalues"="RMS minimum\nvalues", "RMS values"=w189, "Total power values"=w190, "input cluster"=w259, "Blocking in"="R2 Blocking in", "Transfer Trip"=w96) -> ("trip signal"=w45:bool, "Reclose"=→"Relay2 Reclose":bool, "Relay state"=w26:cluster{"Lockout":bool, "State":i16}, "Blocking out"=→"R2 Blocking out":bool[], "output cluster"=w92:T10)  [unwired: 3 in]
    "Relay2 Trip" <- w45
    n153 = feedback-in #7(w92) -> ()
    n154 = feedback #8() -> (w258:T10)  [unwired: 1 in]
    n155 = call "LC_Relay_Protection.vi"("Protection settings"=w303, "Reset Relay"=w25, "RMS minimum\nvalues"="RMS minimum\nvalues", "RMS values"=w158, "Total power values"=w175, "input cluster"=w258, "Blocking in"="R4 Blocking in", "Transfer Trip"=w97) -> ("trip signal"=w47:bool, "Reclose"=→"Relay4 Reclose":bool, "Relay State"=w32:cluster{"Lockout":bool, "State":i16}, "Blocking out"=→"R4 Blocking out":bool[], "output cluster"=w224:T10)  [unwired: 2 in, 1 out]
    "Relay4 Trip" <- w47
    n156 = feedback-in #8(w224) -> ()
    n157 = feedback #9() -> (w260:T10)  [unwired: 1 in]
    n158 = call "LC_Relay_Protection.vi"("Protection settings"=w303, "Reset Relay"=w25, "RMS minimum\nvalues"="RMS minimum\nvalues", "RMS values"=w157, "Total power values"=w228, "input cluster"=w260, "Blocking in"="R3 Blocking in") -> ("trip signal"=w46:bool, "Reclose"=→"Relay3 Reclose":bool, "Relay State"=w33:cluster{"Lockout":bool, "State":i16}, "Blocking out"=→"R3 Blocking out":bool[], "output cluster"=w225:T10)  [unwired: 3 in, 1 out]
    "Relay3 Trip" <- w46
    n159 = feedback-in #9(w225) -> ()
    n160 = local read "R1 Blocking out"() -> (w90:bool[])
    n161 = local read "R2 Blocking out"() -> (w89:bool[])
    n162 = local read "R3 Blocking out"() -> (w88:bool[])
    n163 = local read "R4 Blocking out"() -> (w87:bool[])
    n164 = local read "R5 Blocking out"() -> (w86:bool[])
    n165 = local read "R6 Blocking out"() -> (w85:bool[])
    n166 = local read "R7 Blocking out"() -> (w84:bool[])
    n167 = local read "R8 Blocking out"() -> (w83:bool[])
    n168 = Unbundle By Name(w26) -> ("Lockout"=w27:bool)
    n169 = Unbundle By Name(w28) -> ("Lockout"=w34:bool)
    n170 = feedback #10() -> (w173:cluster{bool, dbl})  [unwired: 1 in]
    n171 = feedback #11() -> (w194:cluster{bool, dbl})  [unwired: 1 in]
    n172 = feedback #12() -> (w184:cluster{bool, dbl})  [unwired: 1 in]
    n173 = feedback #13() -> (w151:cluster{bool, dbl})  [unwired: 1 in]
    n174 = call "LC_Relay_Reclose.vi"("Recloser Settings"="Recloser Settings", "Recloser in"=w194, "Reclose?"="Reclose Relay2?", "VR RMS avg"=w94, "VL RMS avg"=w188, "VR array"=w192, "VL array"=w193) -> ("Phase difference"=w52:dbl, "VR Frequency"=w186:dbl, "VL Frequency"=w187:dbl, "Recloser action"=w246:bool, "Recloser out"=w294:cluster{bool, dbl})
    "Waveform Chart 2" <- w52
    n175 = feedback-in #11(w294) -> ()
    n176 = call "LC_Relay_Reclose.vi"("Recloser Settings"="Recloser Settings", "Recloser in"=w184, "Reclose?"="Reclose Relay3?", "VR RMS avg"=w182, "VL RMS avg"=w183, "VR array"=w180, "VL array"=w181) -> ("Phase difference"=w15:dbl, "VR Frequency"=w16:dbl, "VL Frequency"=w17:dbl, "Recloser action"=w245:bool, "Recloser out"=w185:cluster{bool, dbl})
    n177 = feedback-in #12(w185) -> ()
    n178 = call "LC_Relay_Reclose.vi"("Recloser Settings"="Recloser Settings", "Recloser in"=w173, "Reclose?"="Reclose Relay4?", "VR RMS avg"=w169, "VL RMS avg"=w170, "VR array"=w172, "VL array"=w171) -> ("Phase difference"=w206:dbl, "VR Frequency"=w178:dbl, "VL Frequency"=w177:dbl, "Recloser action"=w244:bool, "Recloser out"=w174:cluster{bool, dbl})
    n179 = feedback-in #10(w174) -> ()
    n180 = call "LC_Relay_Reclose.vi"("Recloser Settings"="Recloser Settings", "Recloser in"=w151, "Reclose?"="Reclose Relay6?", "VR RMS avg"=w149, "VL RMS avg"=w150, "VR array"=w153, "VL array"=w154) -> ("Phase difference"=w276:dbl, "VR Frequency"=w147:dbl, "VL Frequency"=w148:dbl, "Recloser action"=w242:bool, "Recloser out"=w152:cluster{bool, dbl})
    n181 = feedback-in #13(w152) -> ()
    n182 = feedback #14() -> (w133:cluster{bool, dbl})  [unwired: 1 in]
    n183 = call "LC_Relay_Reclose.vi"("Recloser Settings"="Recloser Settings", "Recloser in"=w133, "Reclose?"="Reclose Relay8?", "VR RMS avg"=w131, "VL RMS avg"=w132, "VR array"=w136, "VL array"=w137) -> ("Phase difference"=w266:dbl, "VR Frequency"=w130:dbl, "VL Frequency"=w129:dbl, "Recloser action"=w240:bool, "Recloser out"=w134:cluster{bool, dbl})
    n184 = feedback-in #14(w134) -> ()
    n185 = feedback #15() -> (w202:cluster{bool, dbl})  [unwired: 1 in]
    n186 = call "LC_Relay_Reclose.vi"("Recloser Settings"="Recloser Settings", "Recloser in"=w202, "Reclose?"="Reclose Relay1?", "VR RMS avg"=w198, "VL RMS avg"=w199, "VR array"=w200, "VL array"=w201) -> ("Phase difference"=w53:dbl, "VR Frequency"=w196:dbl, "VL Frequency"=w197:dbl, "Recloser action"=w306:bool, "Recloser out"=w203:cluster{bool, dbl})
    n187 = feedback-in #15(w203) -> ()
    n188 = feedback #16() -> (w118:cluster{bool, dbl})  [unwired: 1 in]
    n189 = call "LC_Relay_Reclose.vi"("Recloser Settings"="Recloser Settings", "Recloser in"=w118, "Reclose?"="Reclose Relay7?", "VR RMS avg"=w141, "VL RMS avg"=w142, "VR array"=w144, "VL array"=w145) -> ("Phase difference"=w298:dbl, "VR Frequency"=w139:dbl, "VL Frequency"=w140:dbl, "Recloser action"=w241:bool, "Recloser out"=w273:cluster{bool, dbl})
    n190 = feedback-in #16(w273) -> ()
    n191 = feedback #17() -> (w167:cluster{bool, dbl})  [unwired: 1 in]
    n192 = call "LC_Relay_Reclose.vi"("Recloser Settings"="Recloser Settings", "Recloser in"=w167, "Reclose?"="Reclose Relay5?", "VR RMS avg"=w93, "VL RMS avg"=w163, "VR array"=w165, "VL array"=w166) -> ("Phase difference"=w282:dbl, "VR Frequency"=w160:dbl, "VL Frequency"=w161:dbl, "Recloser action"=w243:bool, "Recloser out"=w168:cluster{bool, dbl})
    n193 = feedback-in #17(w168) -> ()
    n194 = Unbundle By Name(w29) -> ("Lockout"=w35:bool)
    n195 = Unbundle By Name(w31) -> ("Lockout"=w37:bool)
    n196 = Unbundle By Name(w33) -> ("Lockout"=w39:bool)
    n197 = Unbundle By Name(w30) -> ("Lockout"=w36:bool)
    n198 = Unbundle By Name(w32) -> ("Lockout"=w38:bool)
    n199 = Index Array(array=w138) -> (element #1=w267:dbl, element #2=w268:dbl)  [unwired: 2 in]
    n200 = Unbundle By Name(w40) -> ("Lockout"=w41:bool)
    n201 = Index Array(array=w218) -> (element #1=w263:dbl, element #2=w271:dbl)  [unwired: 2 in]
    n202 = Index Array(array=w219) -> (element #1=w277:dbl, element #2=w278:dbl)  [unwired: 2 in]
    n203 = Index Array(array=w230) -> (element #1=w281:dbl, element #2=w280:dbl)  [unwired: 2 in]
    n204 = Index Array(array=w175) -> (element #1=w287:dbl, element #2=w288:dbl)  [unwired: 2 in]
    n205 = case shown="False" "Manual Relay Control" {
      tunnel: w242 -> [w541 _]
      frame False {
        n206 = local write "Relay6"(w541) -> ()
      }
      frame True {
      }
    }
    n207 = case shown="False" "Manual Relay Control" {
      tunnel: w240 -> [w539 _]
      frame False {
        n208 = local write "Relay8"(w539) -> ()
      }
      frame True {
      }
    }
    n209 = Index Array(array=w190) -> (element #1=w208:dbl, element #2=w207:dbl)  [unwired: 2 in]
    n210 = case shown="False" "Manual Relay Control" {
      tunnel: w243 -> [w542 _]
      frame False {
        n211 = local write "Relay5"(w542) -> ()
      }
      frame True {
      }
    }
    n212 = case shown="False" "Manual Relay Control" {
      tunnel: w241 -> [w540 _]
      frame False {
        n213 = local write "Relay7"(w540) -> ()
      }
      frame True {
      }
    }
    n214 = case shown="False" "Manual Relay Control" {
      tunnel: w306 -> [w607 _]
      frame False {
        n215 = local write "Relay1"(w607) -> ()
      }
      frame True {
      }
    }
    n216 = Index Array(array=w191) -> (element #1=w325:dbl, element #2=w403:dbl)  [unwired: 2 in]
    n217 = case shown="False" "Manual Relay Control" {
      tunnel: w245 -> [w544 _]
      frame False {
        n218 = local write "Relay3"(w544) -> ()
      }
      frame True {
      }
    }
    n219 = Index Array(array=w228) -> (element #1=w285:dbl, element #2=w291:dbl)  [unwired: 2 in]
    n220 = case shown="False" "Manual Relay Control" {
      tunnel: w244 -> [w543 _]
      frame False {
        n221 = local write "Relay4"(w543) -> ()
      }
      frame True {
      }
    }
    n222 = case shown="False" "Manual Relay Control" {
      tunnel: w246 -> [w545 _]
      frame False {
        n223 = local write "Relay2"(w545) -> ()
      }
      frame True {
      }
    }
    n224 = Index Array(array=w90) -> (element #2=w55:bool)  [unwired: 2 in, 1 out]
    n225 = Index Array(array=w89) -> (element #1=w66:bool, element #2=w69:bool)  [unwired: 2 in]
    n226 = Index Array(array=w88) -> (element #2=w78:bool)  [unwired: 2 in, 1 out]
    n227 = Index Array(array=w87) -> (element #1=w79:bool, element #2=w68:bool)  [unwired: 2 in]
    n228 = Index Array(array=w86) -> (element #1=w65:bool, element #2=w82:bool)  [unwired: 2 in]
    n229 = Index Array(array=w85) -> (element #1=w63:bool, element #2=w81:bool)  [unwired: 2 in]
    n230 = Index Array(array=w84) -> (element #1=w64:bool, element #2=w80:bool)  [unwired: 2 in]
    n231 = Index Array(array=w83) -> (element #1=w67:bool)  [unwired: 2 in, 1 out]
    n232 = Subtract(x=w186, y=w187) -> (x-y=w261:dbl)
    n233 = case shown="True" w34 {
      tunnel: [w448 w449] -> w265
      tunnel: w28 -> [_ w450]
      frame False {
        n234 = local read "Relay8"() -> (w447:bool)
        n235 = Boolean To (0,1)(Boolean=w447) -> (0, 1=w448:i16)
      }
      frame True {
        n236 = Unbundle By Name(w450) -> ("State"=w449:i16)
      }
    }
    n237 = Subtract(x=w196, y=w197) -> (x-y=w54:dbl)
    n238 = case shown="True" w35 {
      tunnel: [w443 w445] -> w42
      tunnel: w29 -> [_ w446]
      frame False {
        n239 = local read "Relay7"() -> (w444:bool)
        n240 = Boolean To (0,1)(Boolean=w444) -> (0, 1=w443:i16)
      }
      frame True {
        n241 = Unbundle By Name(w446) -> ("State"=w445:i16)
      }
    }
    n242 = case shown="True" w36 {
      tunnel: [w440 w441] -> w275
      tunnel: w30 -> [_ w442]
      frame False {
        n243 = local read "Relay6"() -> (w439:bool)
        n244 = Boolean To (0,1)(Boolean=w439) -> (0, 1=w440:i16)
      }
      frame True {
        n245 = Unbundle By Name(w442) -> ("State"=w441:i16)
      }
    }
    n246 = case shown="True" w37 {
      tunnel: [w435 w437] -> w283
      tunnel: w31 -> [_ w438]
      frame False {
        n247 = local read "Relay5"() -> (w436:bool)
        n248 = Boolean To (0,1)(Boolean=w436) -> (0, 1=w435:i16)
      }
      frame True {
        n249 = Unbundle By Name(w438) -> ("State"=w437:i16)
      }
    }
    n250 = case shown="True" w39 {
      tunnel: [w427 w429] -> w292
      tunnel: w33 -> [_ w430]
      frame False {
        n251 = local read "Relay3"() -> (w428:bool)
        n252 = Boolean To (0,1)(Boolean=w428) -> (0, 1=w427:i16)
      }
      frame True {
        n253 = Unbundle By Name(w430) -> ("State"=w429:i16)
      }
    }
    n254 = case shown="True" w38 {
      tunnel: [w431 w433] -> w176
      tunnel: w32 -> [_ w434]
      frame False {
        n255 = local read "Relay4"() -> (w432:bool)
        n256 = Boolean To (0,1)(Boolean=w432) -> (0, 1=w431:i16)
      }
      frame True {
        n257 = Unbundle By Name(w434) -> ("State"=w433:i16)
      }
    }
    n258 = case shown="True" w27 {
      tunnel: [w424 w425] -> w296
      tunnel: w26 -> [_ w426]
      frame False {
        n259 = local read "Relay2"() -> (w423:bool)
        n260 = Boolean To (0,1)(Boolean=w423) -> (0, 1=w424:i16)
      }
      frame True {
        n261 = Unbundle By Name(w426) -> ("State"=w425:i16)
      }
    }
    n262 = Build Array(w265, w132, w131, w129, w130, w266, w267, w268, w269, w269) -> (w339:dbl[])
    "R8 Data for\ncommunication" <- w339
    n263 = case shown="True" w41 {
      tunnel: [w419 w421] -> w404
      tunnel: w40 -> [_ w422]
      frame False {
        n264 = local read "Relay1"() -> (w420:bool)
        n265 = Boolean To (0,1)(Boolean=w420) -> (0, 1=w419:i16)
      }
      frame True {
        n266 = Unbundle By Name(w422) -> ("State"=w421:i16)
      }
    }
    n267 = Build Array(w283, w163, w93, w161, w160, w282, w281, w280, w162, w162) -> (w342:dbl[])
    "R5 Data for\ncommunication" <- w342
    n268 = Build Array(w275, w150, w149, w148, w147, w276, w277, w278, w279, w279) -> (w341:dbl[])
    "R6 Data for\ncommunication" <- w341
    n269 = Build Array(w42, w142, w141, w140, w139, w298, w263, w271, w270, w270) -> (w340:dbl[])
    "R7 Data for\ncommunication" <- w340
    n270 = Build Array(w292, w183, w182, w17, w16, w15, w285, w291, w290, w290) -> (w344:dbl[])
    "R3 Data for\ncommunication" <- w344
    n271 = Build Array(w176, w170, w169, w177, w178, w206, w287, w288, w289, w289) -> (w343:dbl[])
    "R4 Data for\ncommunication" <- w343
    n272 = Build Array(w296, w188, w94, w187, w186, w52, w208, w207, 0.0 ("element"), w261) -> (w345:dbl[])
    "R2 Data for\ncommunication" <- w345
    n273 = Build Array(w404, w199, w198, w197, w196, w53, w325, w403, 0.0 ("element"), w54) -> (w346:dbl[])
    "R1 Data for\ncommunication" <- w346
    n274 = Unbundle By Name(w302) -> ("Direction"=w229:enum16{"forward", "backward", "N/D"})
    n275 = Unbundle By Name(w91) -> ("Direction"=w222:enum16{"forward", "backward", "N/D"})
    n276 = Unbundle By Name(w224) -> ("Direction"=w223:enum16{"forward", "backward", "N/D"})
    n277 = Unbundle By Name(w221) -> ("Direction"=w220:enum16{"forward", "backward", "N/D"})
    n278 = Unbundle By Name(w92) -> ("Direction"=w227:enum16{"forward", "backward", "N/D"})
    n279 = Unbundle By Name(w225) -> ("Direction"=w226:enum16{"forward", "backward", "N/D"})
    n280 = Compound Arithmetic op=OR(w78, w66, w79, w65, w63, w64, w67) -> (w77:bool)
    n281 = Compound Arithmetic op=OR(w55, w79, w63, w67, w65, w64) -> (w76:bool)
    n282 = Compound Arithmetic op=OR(w55, w66, w65, w79, w63, w64, w67) -> (w75:bool)
    n283 = Compound Arithmetic op=OR(w55, w69, w63, w78, w67, w65, w64) -> (w74:bool)
    n284 = Compound Arithmetic op=OR(w55, w69, w68, w64, w63, w67, w55) -> (w73:bool)
    n285 = Compound Arithmetic op=OR(w69, w68, w82, w64, w67, w69) -> (w72:bool)
    n286 = Compound Arithmetic op=OR(w68, w82, w81, w67, w69, w55) -> (w71:bool)
    n287 = Compound Arithmetic op=OR(w82, w81, w80, w69, w68) -> (w70:bool)
    n288 = case shown="\"backward\"" w229 {
      tunnel: w44 -> [w537 _]
      frame "forward", Default {
        "R2 Transfer" <- w537
      }
      frame "backward" {
        n289 = local write "R2 Transfer"(FALSE ("R2 Transfer")) -> ()
      }
    }
    n290 = case shown="\"backward\"" w222 {
      tunnel: w48 -> [w529 _]
      frame "forward", Default {
        "R7 Transfer" <- w529
      }
      frame "backward" {
        n291 = local write "R7 Transfer"(FALSE ("R2 Transfer")) -> ()
      }
    }
    n292 = local write "R2 Blocking in"(w76) -> ()
    n293 = local write "R3 Blocking in"(w75) -> ()
    n294 = local write "R4 Blocking in"(w74) -> ()
    n295 = local write "R5 Blocking in"(w73) -> ()
    n296 = local write "R6 Blocking in"(w72) -> ()
    n297 = local write "R7 Blocking in"(w71) -> ()
    n298 = local write "R8 Blocking in"(w70) -> ()
    n299 = local write "R1 Blocking in"(w77) -> ()
    n300 = Subtract(x=w140, y=w139) -> (x-y=w297:dbl)
    n301 = case shown="\"forward\", Default" w223 {
      tunnel: w47 -> [w531 _]
      frame "forward", Default {
        "R5 Transfer" <- w531
      }
      frame "backward" {
        n302 = local write "R5 Transfer"(FALSE ("R2 Transfer")) -> ()
      }
    }
    n303 = case shown="\"forward\", Default" w220 {
      tunnel: w50 -> [w527 _]
      frame "forward", Default {
        "R8 Transfer" <- w527
      }
      frame "backward" {
        n304 = local write "R8 Transfer"(FALSE ("R2 Transfer")) -> ()
      }
    }
    n305 = shared-variable "Relay Control\\LC_Relay_data.lvlib\\f_Relay7_Ang_Diff"(w298) -> ()  [unwired: 1 in, 1 out]
    n306 = case shown="\"forward\", Default" w226 {
      tunnel: w46 -> [w533 _]
      tunnel: [w533 FALSE] -> w300
      frame "forward", Default {
      }
      frame "backward" {
      }
    }
    n307 = shared-variable "Relay Control\\LC_Relay_data.lvlib\\f_Relay7_Freq_Diff"(w297) -> ()  [unwired: 1 in, 1 out]
    n308 = case shown="\"forward\", Default" w227 {
      tunnel: w45 -> [w535 _]
      tunnel: [w535 FALSE] -> w301
      frame "forward", Default {
      }
      frame "backward" {
      }
    }
    n309 = Build Array (concatenate)(w346, w345, w344, w343, w342, w341, w340, w339) -> (w347:dbl[])
    n310 = Or(x=w301, y=w300) -> (x .or. y?=→"R4 Transfer":bool)
    n311 = shared-variable "Relay Control\\LC_Relay_data.lvlib\\ar_Relay_to_MGCC"(w347) -> ()  [unwired: 1 in, 1 out]
    n312 = xnode "Read/Write Control"("FPGA VI Reference In"=w415, "Relay1"="Relay1", "Relay2"="Relay2", "Relay3"="Relay3", "Relay4"="Relay4", "Relay5"="Relay5", "Relay6"="Relay6", "Relay7"="Relay7", "Relay8"="Relay8", "Count(ticks)"="Count(ticks)") -> ("FPGA VI Reference Out"=w417:refnum<k20>, "error out"=w416:errorcluster)  [unwired: 1 in]
    n313 = shared-variable "Relay Control\\LC_Relay_data.lvlib\\b_Relay7_Cmd"("Relay7") -> ()  [unwired: 1 in, 1 out]
    n314 = node-c288() -> ()  [unwired: 1 in, 1 out]
  }
  n315 = node-c288(w3) -> ()  [unwired: 1 out]
  n316 = xnode "Close FPGA VI Reference"("FPGA VI Reference In"=w13, "error in"=w12) -> ()  [unwired: 1 out]
